vi "ExeVersionInformation.vi"(8 "error in (no error)":errorcluster, 11 "path":path) -> (0 "error out":errorcluster, 3 "FileVersion":string)   [LabVIEW 2013, in "main.lvlib"]
uses:
  main.lvlib
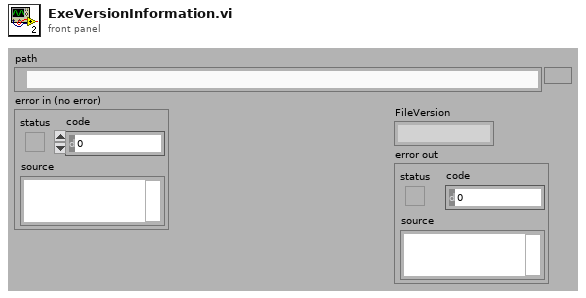
[diagram p1: front panel]
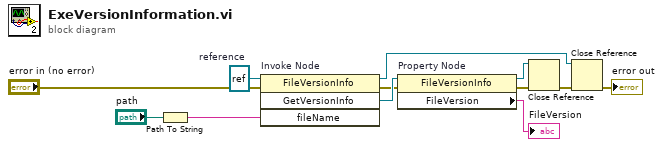
[diagram p0: block diagram]
diagram:
  w12 = refnum<k24> refnum  # reference
  n1 = Path To String(path="path") -> (string=w11:string)
  n2 = invoke on="Invoke Node" class="FileVersionInfo" method="GetVersionInfo"(reference=w12, error in="error in (no error)", "fileName"=w11) -> (reference out=w4:refnum<k24>, error out=w9:errorcluster, "GetVersionInfo"=w10:refnum<k24>)  [unwired: 1 in, 1 out]
  n3 = property on="Property Node" class="FileVersionInfo"(reference=w10, error in=w9) -> (reference out=w7:refnum<k24>, error out=w6:errorcluster, "FileVersion"=→"FileVersion":string)
  n4 = Close Reference(reference=w7, error in (no error)=w6) -> (error out=w5:errorcluster)
  n5 = Close Reference(reference=w4, error in (no error)=w5) -> (error out=→"error out":errorcluster)
